vi "dIMU_Accel.vi"(0 "Maximum Range":enum16{"2g", "4g", "8g"}(ring), 2 "NXT":T2, 3 "Port":T1 items=["Port 1", "Port 2", "Port 3", "Port 4"]) -> (4 "NXT":T2)   [LabVIEW 2010]
uses:
  <vilib>/NXT/Subs/LVHSConnector.ctl
  <vilib>/NXT/Block Support/NXT_InputPort.ctl
  <vilib>/NXT/Block Support/HWPage.SensorType.ctl
  <vilib>/NXT/Block Support/HWPage.SensorMode.ctl
  <vilib>/NXT/Dual Mode Library/Sensors/i2c_sensors.vi
panel:
  out "Array":i32[](array[numeric])
  out "Bytes read":u8[](array[numeric]) format="%.0x"
  out "Divisor":u8
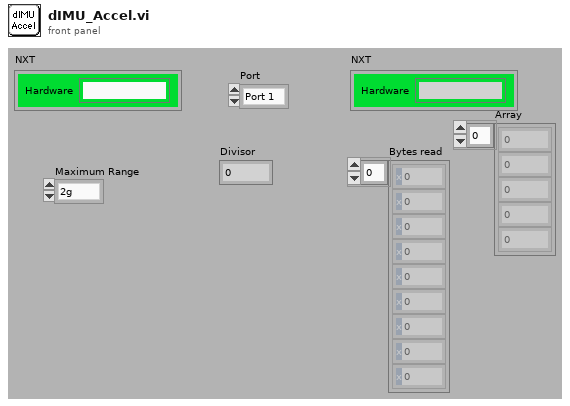
[diagram p1: front panel]
types:
  T1 = typedef "NXT_InputPort.ctl" = u8
  T2 = typedef "LVHSConnector.ctl" = cluster{"Hardware":string, "Flattened String":string}
  T3 = typedef "HWPage.SensorType.ctl" = u8
  T4 = typedef "HWPage.SensorMode.ctl" = u8
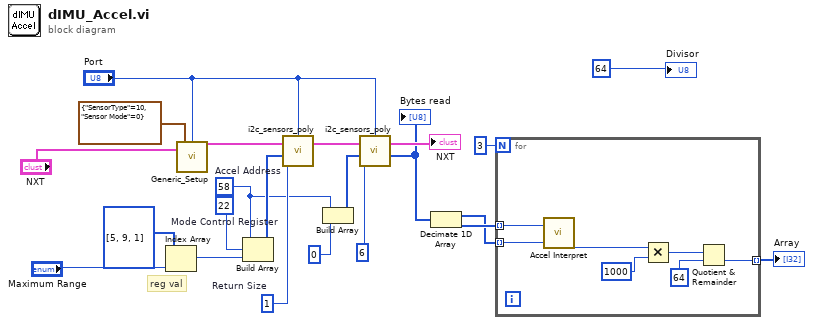
[diagram p0: block diagram]
diagram:
  w8 = u8 58  # Accel Address
  w13 = u8 1  # Return Size
  w16 = i16 22  # Mode Control Register
  # "reg val"
  n1 = Index Array(array=i32[] [5, 9, 1], index="Maximum Range") -> (element=w15:i32)
  n2 = call <vilib>:"Generic_Setup.vi"("Sensor Setup"=cluster{"SensorType":T3, "Sensor Mode":T4} {"SensorType"=10, "Sensor Mode"=0}, "NXT"="NXT", "Port"="Port") -> ("NXT"=w17:T2)  [unwired: 1 out]
  n3 = Build Array(w8, w16, w15) -> (w14:i32[])
  n4 = call-poly <vilib>:"i2c_sensors_poly.vi"("Return Length"=w13, "Bytes to Write"=w14, "NXT"=w17, "Port"="Port") -> ("NXT"=w12:T2)  [unwired: 1 in, 2 out]
  n5 = Build Array(w8, 0) -> (w6:i32[])
  n6 = call-poly <vilib>:"i2c_sensors_poly.vi"("Return Length"=u8 6, "Bytes to Write"=w6, "NXT"=w12, "Port"="Port") -> ("Bytes read"=w5:u8[], "NXT"=→"NXT":T2)  [unwired: 1 in, 1 out]
  "Bytes read" <- w5
  n7 = Decimate 1D Array(w5) -> (w3:u8[], w4:u8[])
  n8 = for {
    N: 3 -> [_]
    tunnel: w4 -> [w29] mode=indexing
    tunnel: w3 -> [w28] mode=indexing
    tunnel: [w23] -> w2 mode=indexing
    n9 = call "Accel Interpret.vi"("LSB"=w28, "MSB"=w29) -> ("Value"=w25:i16)
    n10 = Multiply(x=w25, y=1000) -> (x*y=w26:i32)
    n11 = Quotient & Remainder(x=w26, y=64) -> (floor(x/y)=w23:i32)  [unwired: 1 out]
  }
  "Array" <- w2
  "Divisor" <- 64
